vi "UpdateGaussianFitGraph.vi"(6 "Peak amplitudes":dbl[](array[numeric]), 7 "Best Gaussian Fit":dbl[](array[numeric]), 9 "Peak locations":dbl[](array[numeric]), 10 "Original measured data":cluster{dbl[], dbl[]}, 11 "Control in":refnum<vi>) -> (3 "Control out":refnum<vi>)   [LabVIEW 2013]
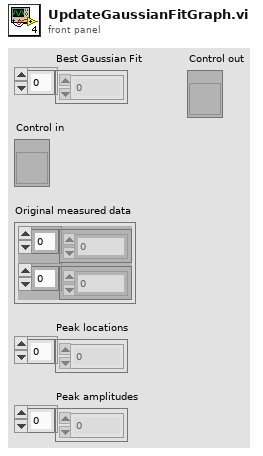
[diagram p1: front panel]
types:
  T1 = cluster{"Peak locations":dbl[], "Peak amplitudes":dbl[]}
  T2 = cluster{"Peak locations":dbl[], "Best Gaussian Fit":dbl[]}
  T3 = cluster{"Peak locations":dbl[], "Best Gaussian Fit":dbl[]}[]
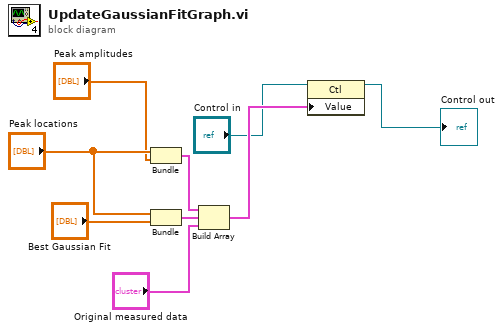
[diagram p0: block diagram]
diagram:
  n1 = Bundle("Peak locations"="Peak locations", "Peak amplitudes"="Peak amplitudes") -> (w7:T1)  [unwired: 1 in]
  n2 = Bundle("Peak locations"="Peak locations", "Best Gaussian Fit"="Best Gaussian Fit") -> (w6:T2)  [unwired: 1 in]
  n3 = Build Array(w7, w6, "Original measured data") -> (w8:T3)
  n4 = property class="Ctl"(reference="Control in", "Value"=w8) -> (reference out=→"Control out":refnum<vi>)  [unwired: 1 in, 1 out]
